vi "FindVar.vi"(8 "error in (no error)":errorcluster, 9 "Tag":string, 10 "Abs_Type Default":refnum<class "Abs_Type.lvclass">, 11 "Var Bus in":refnum<class "Multi_Bus.lvclass">) -> (0 "error out":errorcluster, 2 "Abs_Type Found":refnum<class "Abs_Type.lvclass">, 3 "Var Bus out":refnum<class "Multi_Bus.lvclass">)   [LabVIEW 2021, in "Multi_Bus.lvclass"]
uses:
  Multi_Bus.lvclass
  <vilib>/TSA/Abstract Data Classes/Abs_Types/Type/Abs_Type.lvclass
  <vilib>/TSA/Abstract Data Classes/Abs_Types/Type/Abs_Type.lvclass/Abs_Type.ctl
  Multi_Bus.lvclass/Multi_Bus.ctl
  Properties/Read Var Map.vi
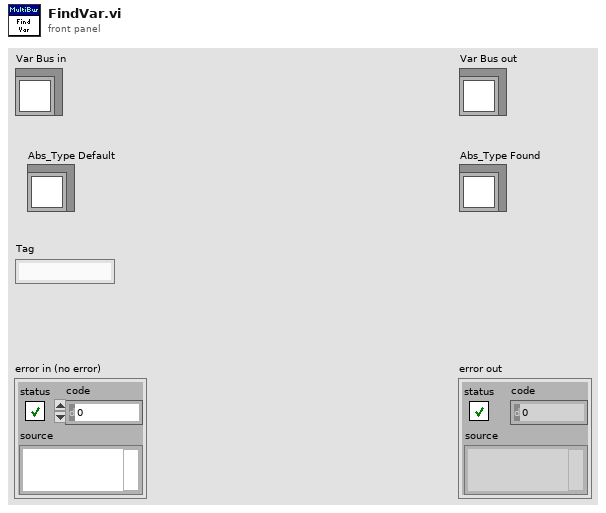
[diagram p1: front panel]
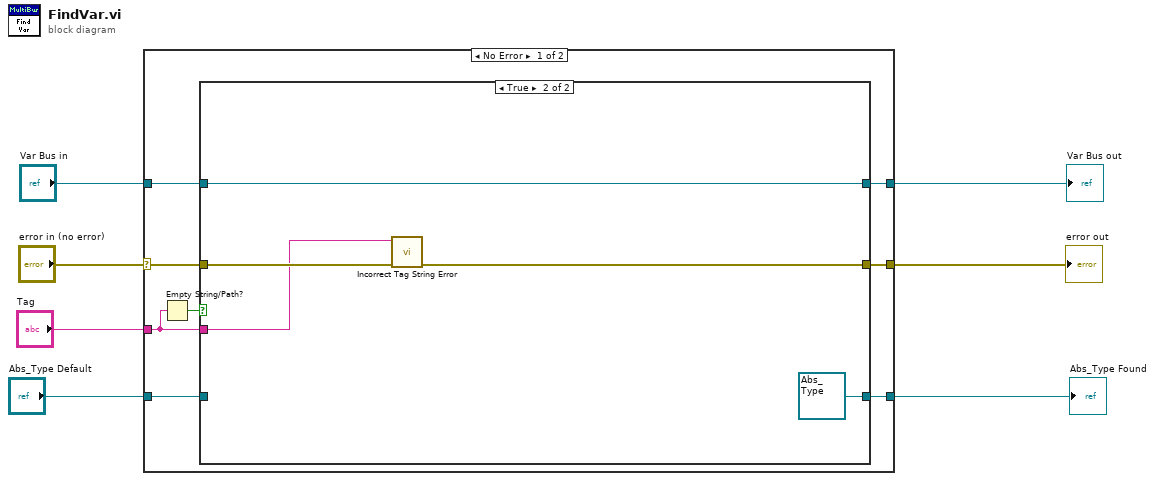
[diagram p0: block diagram]
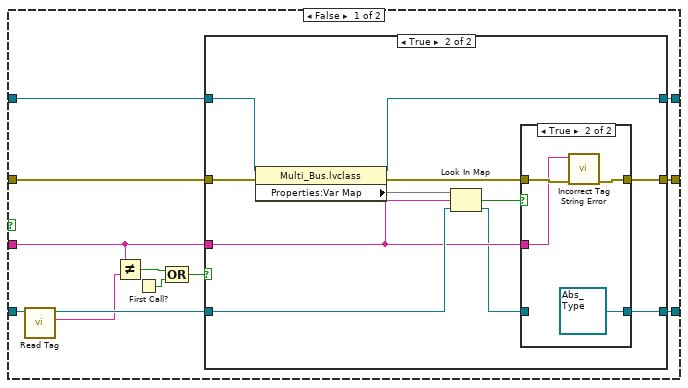
[diagram p2: hidden frame]
diagram:
  n1 = case shown="No Error" "error in (no error)" {
    selector: "error in (no error)" -> [w15 w54]
    tunnel: [w12 w54] -> w6
    tunnel: [w11 w53] -> w4
    tunnel: "Var Bus in" -> [w14 w53]
    tunnel: "Tag" -> [w9 _]
    tunnel: [w13 _] -> w2
    tunnel: "Abs_Type Default" -> [w10 _]
    frame No Error {
      n2 = Empty String/Path?(string/path=w9) -> (empty?=w8:bool)
      n3 = case shown="True" w8 {
        tunnel: w15 -> [w27 w50]
        tunnel: w14 -> [w26 w52]
        tunnel: [w25 refnum<class "Abs_Type.lvclass"> refnum ("Abs_Type.lvclass")] -> w13
        tunnel: [w24 w49] -> w12
        tunnel: [w23 w52] -> w11
        tunnel: w9 -> [w19 w48]
        tunnel: w10 -> [w18 _]
        frame False {
          n4 = call <vilib>:"Read Tag.vi"("Abs_Type in"=w18) -> ("Tag"=w16:string, "Abs_Type out"=w17:refnum<class "Abs_Type.lvclass">)  [unwired: 9 in]
          n5 = Not Equal?(x=w19, y=w16) -> (x != y?=w22:bool)
          n6 = First Call?() -> (First Call?: T/F=w20:bool)
          n7 = Compound Arithmetic op=OR(w22, w20) -> (w21:bool)
          n8 = case shown="True" w21 {
            tunnel: w27 -> [w29 w41]
            tunnel: w26 -> [w28 w40]
            tunnel: [w30 w31] -> w25
            tunnel: [w29 w35] -> w24
            tunnel: [w28 w38] -> w23
            tunnel: w17 -> [w30 w37]
            tunnel: w19 -> [_ w34]
            frame False {
            }
            frame True {
              n9 = property class="Multi_Bus.lvclass"(reference=w40, error in=w41) -> (reference out=w38:refnum<class "Multi_Bus.lvclass">, error out=w36:errorcluster, "Properties:Var Map"=w39:map{string, refnum<class "Abs_Type.lvclass">})
              n10 = Look In Map(map=w39, key=w34, default value=w37) -> (key not found?=w33:bool, value=w32:refnum<class "Abs_Type.lvclass">)
              n11 = case shown="True" w33 {
                tunnel: w36 -> [w43 w47]
                tunnel: [w43 w46] -> w35
                tunnel: w34 -> [_ w45]
                tunnel: w32 -> [w42 _]
                tunnel: [w42 refnum<class "Abs_Type.lvclass"> refnum ("Abs_Type.lvclass")] -> w31
                frame False {
                }
                frame True {
                  n12 = call "Incorrect Tag String Error.vi"("error in (no error)"=w47, "Tag"=w45) -> ("error out"=w46:errorcluster)  [unwired: 9 in]
                }
              }
            }
          }
        }
        frame True {
          n13 = call "Incorrect Tag String Error.vi"("error in (no error)"=w50, "Tag"=w48) -> ("error out"=w49:errorcluster)  [unwired: 9 in]
        }
      }
    }
    frame Error {
    }
  }
  "error out" <- w6
  "Var Bus out" <- w4
  "Abs_Type Found" <- w2
